vi "Get Port.vi"(0 "NXP in":refnum<class "NXP.lvclass">, 5 "VISA resource name":refnum<visa-resource-name>, 9 "Puerto":u8, 11 "error in (no error)":errorcluster) -> (4 "NXP out":refnum<class "NXP.lvclass">, 6 "VISA resource name 2":refnum<visa-resource-name>, 8 "bool response":bool[](array[boolean]), 10 "Response":string, 15 "error out":errorcluster)   [LabVIEW 2020, in "NXP.lvclass"]
uses:
  NXP.lvclass
  33c1054d-ef18-4202-a1f7-e125606b0dab.vi
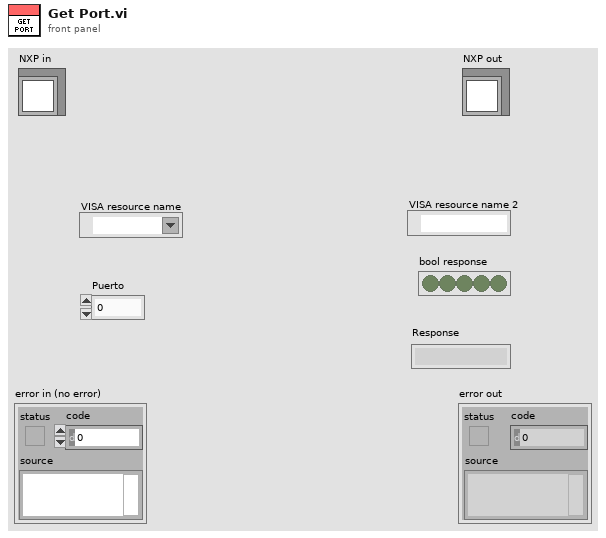
[diagram p1: front panel]
types:
  T1 = enum16{"Write", "Read", "Config", "Reset", "Close"}
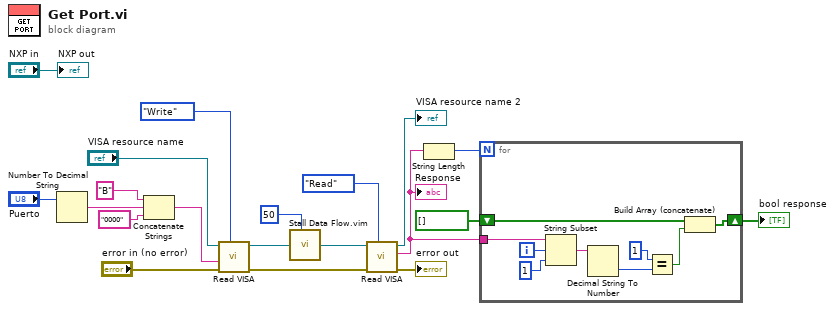
[diagram p0: block diagram]
diagram:
  n1 = Number To Decimal String(number="Puerto") -> (decimal integer string=w15:string)  [unwired: 1 in]
  n2 = Concatenate Strings("B" ("string"), w15, "0000" ("string")) -> (w16:string)
  n3 = call "Read VISA.vi"("Opciones"=T1."Write", "error in (no error)"="error in (no error)", "Write"=w16, "VISA com port"="VISA resource name") -> ("error out"=w10:errorcluster, "VISA com port 2"=w13:refnum<visa-resource-name>)  [unwired: 5 in, 1 out]
  n4 = call "Stall Data Flow.vim"("value in"=w13, "milliseconds to wait"=u32 50) -> ("value out"=w12:refnum<visa-resource-name>)  [unwired: 1 out]
  n5 = call "Read VISA.vi"("Opciones"=T1."Read", "error in (no error)"=w10, "VISA com port"=w12) -> ("error out"=→"error out":errorcluster, "Read"=w4:string, "VISA com port 2"=→"VISA resource name 2":refnum<visa-resource-name>)  [unwired: 6 in]
  "Response" <- w4
  n6 = String Length(string=w4) -> (length=w3:i32)
  n7 = for {
    N: w3 -> [_]
    tunnel: w4 -> [w29]
    shift-right: [w22] -> w5
    shift-left: bool[] [] -> [w21]
    i -> [w28]
    n8 = String Subset(string=w29, offset (0)=w28, length (rest)=1 ("length (rest)")) -> (substring=w26:string)
    n9 = Decimal String To Number(string=w26) -> (number=w25:i32)  [unwired: 2 in, 1 out]
    n10 = Equal?(x=1, y=w25) -> (x = y?=w23:bool)
    n11 = Build Array (concatenate)(w21, w23) -> (w22:bool[])
  }
  "bool response" <- w5
  "NXP out" <- "NXP in"
